vi "NonVILib Single String To Qualified Name Array.vi"(1 "Fully Qualified String":string) -> (0 "Fully Qualified Array":string[](array[string]))   [LabVIEW 2010]
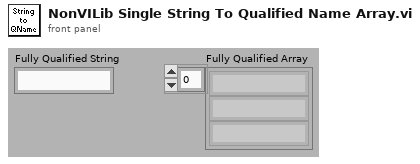
[diagram p1: front panel]
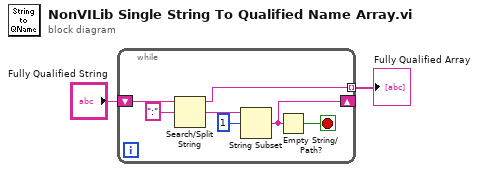
[diagram p0: block diagram]
diagram:
  n1 = while {
    tunnel: [w7] -> w2 mode=indexing
    shift-right: [w4] -> _
    shift-left: "Fully Qualified String" -> [w9]
    stop <- w3 stop-if-true
    n2 = Search/Split String(string=w9, search string/char (-)=":") -> (substring before match=w7:string, match + rest of string=w6:string)  [unwired: 1 in, 1 out]
    n3 = String Subset(string=w6, offset (0)=1) -> (substring=w4:string)  [unwired: 1 in]
    n4 = Empty String/Path?(string/path=w4) -> (empty?=w3:bool)
  }
  "Fully Qualified Array" <- w2
